vi "AlliGator FLI Dataset Series Actions.vi"(0 "AlliGator Q Elements":T4[](array[typedef]), 1 "VI in":refnum<vi>, 2 "Script in":bool, 5 "AlliGator IV DVR in":refnum<data-value>, 7 "AlliGator Q Event in":T5=enum."GUI:Idle", 9 "Data":variant, 11 "error in (no error)":errorcluster, 12 "AlliGator Ctrl Refnums":T6) -> (3 "Script out":bool, 4 "Alligator Queue Elements":T4[](array[typedef]), 6 "AlliGator IV DVR out":refnum<data-value>, 10 "[Notebook Message]":T1[](array[typedef]) {"Message Style"."Text Alignment" items=["Left", "Right", "Center"]}, 15 "error out":errorcluster)   [LabVIEW 2021, in "AlliGator Action Engine.lvlib"]
doc: "Processes AlliGator FLI Dataset Series-related actions."
uses:
  AlliGator Action Engine.lvlib
  AlliGator Internal Variables v2.ctl
  <vilib>/vision/Image Controls.llb/IMAQ Image.ctl
  AlliGator Gate Image Set.ctl
  AlliGator FLI Dataset Type.ctl
  AlliGator Data Series Type.ctl
  AlliGator Dataset Channel.ctl
  AlliGator Gate Arithmetic.ctl
  AlliGator Displayed Image.ctl
  Image/Named ROI Description.ctl
  AlliGator Decay Metadata v3.ctl
  AlliGator Decay Background Subtraction Info.ctl
  AlliGator Baseline Subtraction Method.ctl
  Graphs/XY Graph/XY Graph Plot Shift Parameters.ctl
  Graphs/XY Graph/XY Graph Plot Shift Method.ctl
  AlliGator Decay Extrapolation Parameters.ctl
  Phasor/Calibration Phasor (m, phi).ctl
  Phasor/Phasor Reference Series.ctl
  Phasor/Phasor Calibration Map v2.ctl
  Phasor/Phasor (g, s).ctl
  AlliGator Raw Phasor Plot Data v4.ctl
  Phasor/Phasor Standard Deviation Options.ctl
  AlliGator Phasor Multi-Harmonic Data.ctl
  Phasor/Phasor Harmonic Data.ctl
  AlliGator Decay Fit Options & Parameters v2.ctl
  Fits/IRF(X)PSED/Decay Fit Options v2.ctl
  Fits/Decay Convolution/Decay Model.ctl
  Fits/Residual Type.ctl
  Fits/IRF(X)PSED/Fit Weights Type.ctl
  Fits/Non-linear Fitting Method v2.ctl
  Fits/Fit Calculation Method.ctl
  Fits/Non-linear Fitting Algorithm.ctl
  AlliGator Decay Fit Parameter Constraints 2.ctl
  Fits/IRF(X)PSED/Decay Fit Parameters In List.ctl
  Fits/IRF(X)PSED/MLE Baseline Offset Type.ctl
  AlliGator Decay Preprocessing Parameters.ctl
  Fits/IRF(X)PSED/Decay Fit Parameters & Derived Quantities List.ctl
  AlliGator Q Event.ctl
  AlliGator Ctrl Refnums.ctl
  AlliGator Other Ctrl Refnums.ctl
  AlliGator State Indicator.ctl
  AlliGator Phasor Plot Ctrl Refnums.ctl
  AlliGator Phasor Graph Ctrl Refnums.ctl
  Phasor/Phasor Calibration Type.ctl
  AlliGator Dataset Ctrl Refnums.ctl
  AlliGator Registered Events Ctrl Refnums.ctl
  AlliGator Image Histogram Control Refnums.ctl
  Histograms/Linear Histogram Options.ctl
  Histograms/Histogram Bin Option.ctl
  Histograms/Histogram Bin Position.ctl
  AlliGator Decay Fit Map Control Refnums.ctl
  AlliGator Q Element.ctl
  Notebook/Notebook Message Object.ctl
  Rich Text Box/Text Formatting.ctl
  Rich Text Box/Text Colors.ctl
  Alligator Elements Order in Action Stack.ctl
  AlliGator Variables List.ctl
  AlliGator Series Analysis Type.ctl
  AlliGator Globals.vi
  Variant/Variant to Data/Variant to DBL.vi
  Variant/Variant to Data/Variant to Boolean.vi
  AlliGator Add Action Array to Stack.vi
  GUI/GUI.lvlib
  AlliGator Accumulated Dataset.lvlib
  AlliGator Scripts.lvlib
  Sound/Sound.lvlib
  AlliGator Decay Fit.lvlib
  AlliGator Internal Variables.lvlib
  Image/Image.lvlib
  Variant/Variant to Data/Variant to Data.lvlib
  AlliGator Source Image.lvlib
  AlliGator Globals, Variables & Constants.lvlib
  Rich Text Box/Rich Text Box.lvlib
  Phasor/Phasor.lvlib
  AlliGator Decay Preprocessing.lvlib
  Graphs/XY Graph/XY Graph Add-Ons.lvlib
  AlliGator Phasor Graph.lvlib
  AlliGator Files.lvlib
  AlliGator Phasor Plot.lvlib
  Fits/Fits.lvlib
  AlliGator Decay Fit Parameter Map.lvlib
  AlliGator Settings.lvlib
  AlliGator GUI.lvlib
  AlliGator Dual-Channel Datasets.lvlib
  Histograms/Histogram Window.lvlib
  Notebook/Notebook.lvlib
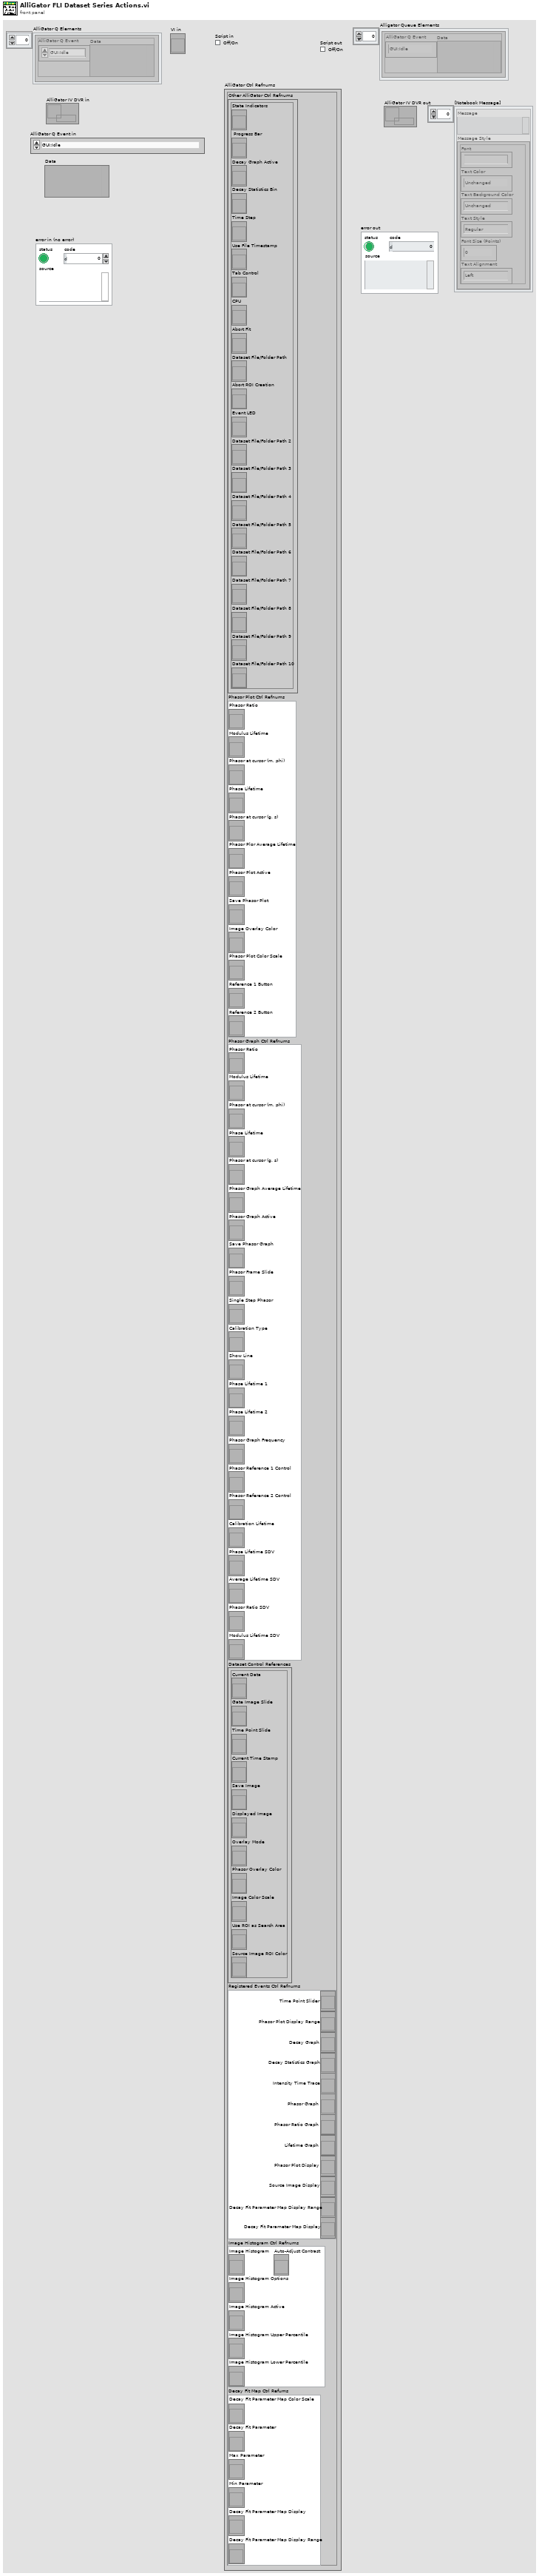
[diagram p1: front panel]
types:
  T1 = typedef "Notebook.lvlib/Notebook Message Object.ctl" = cluster{"Message":string, "Message Style":T2}
  T2 = typedef "Rich Text Box.lvlib/Text Formatting.ctl" = cluster{"Font":string, "Text Color":T3, "Text Background Color":T3, "Text Style":enum16{"Regular", "Bold", "Italic", "Underline", "Strikeout"}, "Font Size (Points)":dbl, "Text Alignment":i32}
  T3 = typedef "Rich Text Box.lvlib/Text Colors.ctl" = enum16{"Unchanged", "Black", "Blue", "Brown", "Gray", "Green", "Orange", "Pink", "Red", "White"}
  T4 = typedef "AlliGator Action Engine.lvlib/AlliGator Q Element.ctl" = cluster{"AlliGator Q Event":T5, "Data":variant}
  T5 = typedef "AlliGator Action Engine.lvlib/AlliGator Q Event.ctl" = enum16{"---- Files ----", "Files:Set Batch Export Files To Save", "Files:Set Dataset Loading & Pre-processing Options", "Files:Check #Frames in Dataset", "Files:Increment Frame Index", "Files:Open Mask Image", "Files:Open White Light Image", "Files:Open Single Dataset", "Files:New Folder of Folders Selected", "Files:Load File (all Types)_Scriptable", "Files:Move Flattened Series to Folders Series", "Files:Select Folder", "Files:Load FLI Dataset", "Files:Load Swiss SPAD 1 Dataset", "Files:Load Swiss SPAD 2 Dataset", "Files:Load .sdt FLI Dataset", "Files:Load .ptu FLI Dataset", "Files:Load .bin FLI Dataset", "Files:Load Single Gate Image Folder", "Files:Load I/m/phi Dataset (deprecated)", "Files:Load Single Image", "Files:Subtract Background File", "Files:Export FLI Dataset", "Files:Load HDF5 FLI Dataset", "Files:Set Destination File Path", "Files:Save Mask Image", "Files:Batch Conversion", "Files:New Folder Selected", "Files:Close FLI Dataset", "Files:Close FLI Dataset Series", "Files:Close White Light Image", "Files:Close Mask Image", "---- FLI Dataset ----", "FLI Dataset:Channel Arithmetic", "FLI Dataset:Export Average Lifetime Map as ASCII", "FLI Dataset:Export User-Defined Quantity Map as ASCII", "FLI Dataset:Python Function FLI Dataset Event", "FLI Dataset:ROI Analysis", "FLI Dataset:Tilted Logistic Square Gated IRF Characteristics Map", "FLI Dataset:Logistic Square Gated IRF Characteristics Map", "FLI Dataset:Square Gated IRF Characteristics Map", "FLI Dataset:Multi-ROI Single-Pixel Phasor Analysis", "FLI Dataset:Multi-ROI Single-Pixel NLSF Analysis", "FLI Dataset:All ROIs IRF Extraction", "FLI Dataset:All ROIs Decay Fit Non-Interactive (Fast + Individual IRF)", "FLI Dataset:All ROIs Phasor Analysis", "FLI Dataset:All ROIs Decay Fit", "FLI Dataset:Fluorescence Decay Statistics", "FLI Dataset:Update Decay Statistics Graph", "FLI Dataset:Get Decay from ROI", "FLI Dataset:All ROIs Average Lifetimes", "---- FLI Dataset Series ----", "FLI Dataset Series:Sum All Datasets in Series", "FLI Dataset Series:Add Dataset to Accumulated Dataset", "FLI Dataset Series:Display Accumulated Dataset", "FLI Dataset Series:Clear Dataset Series Sum", "FLI Dataset Series:Time-Series Analysis (NLSF)", "FLI Dataset Series:Time-Series Analysis (Phasor)", "---- Image ----", "Image:Update Image Profile Plots", "Image:Image Histogram Cursor Move", "Image:Image Histogram", "Image:Image Contrast", "Image:Set Image Histogram Cursor Move Flag", "Image:Clear Image Overlay", "Image:Use ROI as Search Area", "Image:Set ROI Diameter", "Image:Save Image Data as TIFF", "Image:Save Displayed Image with Overlay", "Image:Save Image Overlay Only", "Image:Save Image as Hot Pixel Mask", "Image:Change Source Image Color Palette", "Image:Copy Image to Clipboard", "Image:Source Image ROI Selection", "Image:Delete All ROIs", "Image:Delete All Unselected ROIs", "Image:Delete ROI", "Image:Merge All ROIs", "Image:Store ROI", "Image:Source Image ROI Storage", "Image:Export ROI Description to Notebook", "Image:Save ROI", "Image:Load ROI", "Image:Paste ROI Definition", "Image:Clear ROI", "Image:Identify ROIs in Mask Image", "Image:Create Complementary ROI", "Image:Create Contour ROI", "Image:Create ROI(s) from Pixels with Peak above Min_Scriptable", "Image:Create ROI(s) from Pixels with Intensity above Min_Scriptable", "Image:Compute ROI Statistics", "Image:Delete ROI(s) based on ROI Characteristics", "Image:Create ROI Grid", "Image:ROI to Individual Pixel ROIs", "Image:Python Function Source Image Event", "Image:Show Phasor Calibration Map ROI Centers", "Image:Convert ROI to Mask Image", "Image:Mouse Move", "Image:Mouse Up", "Image:Set Source Image Mouse Move Flag", "Image:Add Scale Bar Overlay", "Image:Delete Existing ROIs Option", "---- Decay ----", "Decay:Clear IRF/Reference Plot", "Decay:Clear Local IRFs", "Decay:Add Decay to Graph", "Decay:Smoothen Plot", "Decay:Smoothen Plot Tail", "Decay:Average Selected Plots", "Decay:Extract IRF", "Decay:Optimal IRF Extraction", "Decay:Threshold IRF", "Decay:Fit to Model IRF", "Decay:Fit IRF to Square Gate", "Decay:Fit IRF to Logistic Square Gate", "Decay:Fit IRF to Tilted Logistic Square Gate", "Decay:Create Bounding Cursors Set", "Decay:Export Bounding Cursors Definition to Notebook", "Decay:Denoise Plot", "Decay:Compute Cumulative Function", "Decay:Use as Reference Decay", "Decay:Show Reference Decay/IRF", "Decay:Extrapolate Decay", "Decay:Create Head & Tail Bounding Cursors", "Decay:Store Cursor-defined Head & Tail Fractions", "Decay:Rebin Plot", "Decay:1-Normalize Decay", "Decay:[0-1]-Normalize Plot", "Decay:Straighten Decay", "Decay:Shift Decay", "Decay:Fold Decay", "Decay:Fit Decay", "Decay:Global Fit of Selected Decays", "Decay:Post Global Fit Script", "Decay:Add Global Fit Parameters to Graph", "Decay:Add Decay Parameter(s) to Plot (Graph)", "Decay:Export Decay to Phasor Graph", "Decay:Plot Decay Shifts", "Decay:Compute Average Lifetime", "Decay:Plot Convolution", "Decay:Graph Tip Strip Update", "---- Decay Statistics ----", "Decay Statistics:Tip Strip Update", "---- Intensity Time Trace ----", "Intensity Time Trace:Use File Timestamp", "Intensity Time Trace:Load Intensity Corrections File", "Intensity Time Trace:Clear Intensity Corrections File", "Intensity Time Trace:Tip Strip Update", "---- Phasor Plot ----", "Phasor Plot:Build Phasor Plot", "Phasor Plot:Change Phasor Plot Color Palette", "Phasor Plot:Adjust Phasor Plot Display Range", "Phasor Plot:Highlight Image ROI in Phasor Plot", "Phasor Plot:Save Phasor Plot Image with Overlay", "Phasor Plot:Export Complex Phasor Map", "Phasor Plot:Export Phasor Ratio Map", "Phasor Plot:Export Average Lifetime Map", "Phasor Plot:Compute Phase Lifetime Histogram", "Phasor Plot:Compute Phasor Ratio Histogram", "Phasor Plot:Compute Phase Lifetime vs Intensity Scatter Plot", "Phasor Plot:Weber 2-Component Decomposition", "Phasor Plot:Update Phasor Color Map Vertices", "Phasor Plot:Clear Phasor Overlay", "Phasor Plot:Use Segment Extremities as References", "Phasor Plot:Use UC/Segment Intersections as References", "Phasor Plot:Use UC/Principal Axis Intersections as References", "Phasor Plot:Use UC/Linear Fit Intersections as References", "Phasor Plot:Update Phasor Plot Reference", "Phasor Plot:Show Local Phasor Info in Phasor Plot", "Phasor Plot:Update Phasor Plot State", "Phasor Plot:Phasor Plot ROI Storage", "Phasor Plot:Phasor Plot ROI Selection", "Phasor Plot:Python Function Phasor Plot Event", "Phasor Plot:Overlay Phasor ROI, Ratio or Map in Source Image", "Phasor Plot:Compute Decay of Selected Phasors", "Phasor Plot:Phasor at Image Pixel", "Phasor Plot:Mouse Move", "Phasor Plot:Mouse Up", "Phasor Plot:Display Range Mouse Move", "Phasor Plot:Set Mouse Move Flag", "---- Phasor Graph ----", "Phasor Graph:Calibrated Phasor Map Series", "Phasor Graph:Whole Image Phasor Scatter Plot (Todo)", "Phasor Graph:Get Phasor Value", "Phasor Graph:Create New Phasor Plot Dialog", "Phasor Graph:Update Last Phasor Value", "Phasor Graph:Update Phasor (m, phi)", "Phasor Graph:Remove Single Phasor from Plot", "Phasor Graph:Add Single Phasor to Plot", "Phasor Graph:Remove Phasor Plot", "Phasor Graph:Remove Selected Phasor Plots", "Phasor Graph:Clear Phasor Data", "Phasor Graph:Clear Phasor Graph", "Phasor Graph:Cursor Move", "Phasor Graph:Draw Cursor Connecting Line", "Phasor Graph:Clear Cursor Connecting Line", "Phasor Graph:Find UC Intersection", "Phasor Graph:Use UC/Cursor-Defined Line Intersections", "Phasor Graph:Use Selected Plots Fitted Line/UC Intersections", "Phasor Graph:Use Selected Plots Principal Axis/UC Intersections", "Phasor Graph:Show Single Phasor", "Phasor Graph:Save Single Phasor Plot", "Phasor Graph:Save All Phasor Plots", "Phasor Graph:Load Phasor Plot(s)", "Phasor Graph:Phasor Multiplication", "Phasor Graph:Compute Average Phasor", "Phasor Graph:Compute Multiple Average Phasors (Selected Plots)", "Phasor Graph:Export Single Phasor Plot Phase Lifetimes", "Phasor Graph:Phase Lifetime Trajectory", "Phasor Graph:Phase Lifetime vs Intensity Scatter Plot (deprecated)", "Phasor Graph:Parameter 2 vs Parameter 1 Scatter Plot", "Phasor Graph:Use Cursor n Location", "Phasor Graph:Set Reference n to Current Phase Lifetime Value", "Phasor Graph:Set Reference n to Lifetime Value", "Phasor Graph:Set Cursor n Location", "Phasor Graph:Save Phasor Graph Image", "Phasor Graph:Update SEPL Plot", "Phasor Graph:Export Single Phasor Plot Data", "Phasor Graph:Export Selected Phasor Plots Data", "Phasor Graph:Python Function Phasor Graph Event", "Phasor Graph:Tip Strip Update", "---- Calibration ----", "Calibration:Set Calibration Type", "Calibration:Load/Save Phasor Calibration", "Calibration:Load/Save Phasor Calibration Series", "Calibration:Load/Save Phasor Calibration Map", "Calibration:Use as Calibration", "Calibration:Compute Optimal Calibration from Phasor References", "Calibration:Clear Phasor Calibration", "Calibration:Single Phasor Calibration Information", "Calibration:Use as Calibration Series", "Calibration:Use as Calibration Map", "Calibration:Clear Calibration Series", "Calibration:Phasor Calibration Series Information", "Calibration:Clear Calibration Map", "Calibration:Phasor Calibration Map Information", "Calibration:Apply Phasor Calibration", "Calibration:Update Single Plot Calibration", "Calibration:Update Multiple Plots Calibration", "Calibration:Clear Single Plot Calibration", "Calibration:Clear All Plots Calibrations", "Calibration:Clear Plot(s) Calibration(s)?", "Calibration:Phasor Calibration Maps (# Gates Series)", "---- Phasor Ratio ----", "Phasor Ratio:Clear Reference n", "Phasor Ratio:Toggle Selected Plot(s)  Lock to Reference 1", "Phasor Ratio:Use as Reference n", "Phasor Ratio:Send Reference n to Notebook", "Phasor Ratio:Toggle Selected Plot(s)  Lock to Reference 2", "Phasor Ratio:Compute Phasor Ratio at Mouse Location", "Phasor Ratio:Compute Phasor Plot's Average Phasor Ratio", "Phasor Ratio:Compute Time-Series Phasor Ratios", "Phasor Ratio:Fit Line to Phasor Ratio Plot", "Phasor Ratio:Save References", "Phasor Ratio:Load References", "Phasor Ratio:Update Phasor Reference 1", "Phasor Ratio:Update Phasor Reference 2", "Phasor Ratio:Move Cursor n to Reference n", "Phasor Ratio:Use as Phasor Reference 1 Lifetime", "Phasor Ratio:Use as Phasor Reference 2 Lifetime", "Phasor Ratio:Export Phasor Ratio Map as ASCII", "Phasor Ratio:Tip Strip Update", "---- Lifetime & Other Parameters Graph ----", "Lifetime:Tip Strip Update", "---- Decay Fit Parameter Map ----", "Decay Fit Parameter Map:Export ROI NLSF Data as ASCII", "Decay Fit Parameter Map:Set Decay Fit  Parameter Map Selection", "Decay Fit Parameter Map:Build Decay Fit Parameter Map", "Decay Fit Parameter Map:Change Decay Fit Parameter Map Color Palette", "Decay Fit Parameter Map:Export Decay Fit Parameter Map Data as ASCII", "Decay Fit Parameter Map:Export All Decay Fit Parameter Maps Data as ASCII", "Decay Fit Parameter Map:Send Map Data to Lifetime Graph", "Decay Fit Parameter Map:Save Decay Fit Parameter Map Image", "Decay Fit Parameter Map:Save-Load IRFs & Fit Data", "Decay Fit Parameter Map:Update Local Decay Plots", "Decay Fit Parameter Map:Python Function Decay Fit Parameters Map Event", "Decay Fit Parameter Map:Overlay Decay Fit Parameter Map in Source Image", "Decay Fit Parameter Map:Plot Map Data vs Intensity", "Decay Fit Parameter Map:Mouse Up", "Decay Fit Parameter Map:Display Range Mouse Move", "---- Generic Graph ----", "Generic Graph:Generic XY Graph Event", "Generic Graph:Python Function XY Graph Event", "Generic Graph:New Plot", "Generic Graph:Save Plot", "Generic Graph:XY Plot Histogram", "Generic Graph:Set XY Graph Plot Name", "Generic Graph:Set Last Cursor Style", "Generic Graph:Tip Strip Update", "---- GUI ----", "GUI:Start Script", "GUI:Type of Displayed Image Changed", "GUI:Gate Image Slide Changed", "GUI:Show Busy Icon", "GUI:Show Busy Icon & Abort Button", "GUI:Hide Busy Icon", "GUI:Hide Busy Icon & Abort Button", "GUI:Abort", "GUI:End Script", "GUI:Start Timing", "GUI:End Timing", "GUI:Set State Indicator", "GUI:Send Parameters JSON Strings to Clipboard", "GUI:Set Gate Step", "GUI:Idle", "GUI:Initialization", "GUI:Quit", "GUI:Increment Dataset Index", "GUI:Set Dataset Index to -1", "GUI:Time Series Slider Moved", "GUI:Time Series Slider Changed", "GUI:Toggle Playback or Loop", "GUI:Playback Script", "GUI:Set Phasor Frequency", "GUI:Open Window", "GUI:Start Test Script", "GUI:End Test Script", "DEBUG"}
  T6 = typedef "AlliGator GUI.lvlib/AlliGator Ctrl Refnums.ctl" = cluster{"Other AlliGator Ctrl Refnums":T7, "Phasor Plot Ctrl Refnums":T8, "Phasor Graph Ctrl Refnums":T9, "Dataset Control References":T10, "Registered Events Ctrl Refnums":T11, "Image Histogram Ctrl Refnums":T12, "Decay Fit Map Ctrl Refums":T13}
  T7 = typedef "AlliGator GUI.lvlib/AlliGator Other Ctrl Refnums.ctl" = cluster{"State Indicators":refnum<vi>, " Progress Bar":refnum<vi>, "Decay Graph Active":refnum<vi>, "Decay Statistics Bin":refnum<vi>, "Time Step":refnum<vi>, "Use File Timestamp":refnum<vi>, "Tab Control":refnum<vi>, "CPU":refnum<vi>, "Abort Fit":refnum<vi>, "Dataset File/Folder Path":refnum<vi>, "Abort ROI Creation":refnum<vi>, "Event LED":refnum<vi>, "Dataset File/Folder Path 2":refnum<vi>, "Dataset File/Folder Path 3":refnum<vi>, "Dataset File/Folder Path 4":refnum<vi>, "Dataset File/Folder Path 5":refnum<vi>, "Dataset File/Folder Path 6":refnum<vi>, "Dataset File/Folder Path 7":refnum<vi>, "Dataset File/Folder Path 8":refnum<vi>, "Dataset File/Folder Path 9":refnum<vi>, "Dataset File/Folder Path 10":refnum<vi>}
  T8 = typedef "AlliGator GUI.lvlib/AlliGator Phasor Plot Ctrl Refnums.ctl" = cluster{"Phasor Ratio":refnum<vi>, "Modulus Lifetime":refnum<vi>, "Phasor at cursor (m, phi)":refnum<vi>, "Phase Lifetime":refnum<vi>, "Phasor at cursor (g, s)":refnum<vi>, "Phasor Plor Average Lifetime":refnum<vi>, "Phasor Plot Active":refnum<vi>, "Save Phasor Plot":refnum<vi>, "Image Overlay Color":refnum<vi>, "Phasor Plot Color Scale":refnum<vi>, "Reference 1 Button":refnum<vi>, "Reference 2 Button":refnum<vi>}
  T9 = typedef "AlliGator GUI.lvlib/AlliGator Phasor Graph Ctrl Refnums.ctl" = cluster{"Phasor Ratio":refnum<vi>, "Modulus Lifetime":refnum<vi>, "Phasor at cursor (m, phi)":refnum<vi>, "Phase Lifetime":refnum<vi>, "Phasor at cursor (g, s)":refnum<vi>, "Phasor Graph Average Lifetime":refnum<vi>, "Phasor Graph Active":refnum<vi>, "Save Phasor Graph":refnum<vi>, "Phasor Frame Slide":refnum<vi>, "Single Step Phasor":refnum<vi>, "Calibration Type":refnum<vi>, "Show Line":refnum<vi>, "Phase Lifetime 1":refnum<vi>, "Phase Lifetime 2":refnum<vi>, "Phasor Graph Frequency":refnum<vi>, "Phasor Reference 1 Control":refnum<vi>, "Phasor Reference 2 Control":refnum<vi>, "Calibration Lifetime":refnum<vi>, "Phase Lifetime SDV":refnum<vi>, "Average Lifetime SDV":refnum<vi>, "Phasor Ratio SDV":refnum<vi>, "Modulus Lifetime SDV":refnum<vi>}
  T10 = typedef "AlliGator GUI.lvlib/AlliGator Dataset Ctrl Refnums.ctl" = cluster{"Current Data":refnum<vi>, "Gate Image Slide":refnum<vi>, "Time Point Slide":refnum<vi>, "Current Time Stamp":refnum<vi>, "Save Image":refnum<vi>, "Displayed Image":refnum<vi>, "Overlay Mode":refnum<vi>, "Phasor Overlay Color":refnum<vi>, "Image Color Scale":refnum<vi>, "Use ROI as Search Area":refnum<vi>, "Source Image ROI Color":refnum<vi>}
  T11 = typedef "AlliGator GUI.lvlib/AlliGator Registered Events Ctrl Refnums.ctl" = cluster{"Time Point Slider":refnum<vi>, "Phasor Plot Display Range":refnum<vi>, "Decay Graph":refnum<vi>, "Decay Statistics Graph":refnum<vi>, "Intensity Time Trace":refnum<vi>, "Phasor Graph":refnum<vi>, "Phasor Ratio Graph":refnum<vi>, "Lifetime Graph":refnum<vi>, "Phasor Plot Display":refnum<vi>, "Source Image Display":refnum<vi>, "Decay Fit Parameter Map Display Range":refnum<vi>, "Decay Fit Parameter Map Display":refnum<vi>}
  T12 = typedef "AlliGator GUI.lvlib/AlliGator Image Histogram Control Refnums.ctl" = cluster{"Image Histogram":refnum<vi>, "Image Histogram Options":refnum<vi>, "Image Histogram Active":refnum<vi>, "Image Histogram Upper Percentile":refnum<vi>, "Image Histogram Lower Percentile":refnum<vi>, "Auto-Adjust Contrast":refnum<vi>}
  T13 = typedef "AlliGator Decay Fit Parameter Map.lvlib/AlliGator Decay Fit Map Control Refnums.ctl" = cluster{"Decay Fit Parameter Map Color Scale":refnum<vi>, "Decay Fit Parameter":refnum<vi>, "Max Parameter":refnum<vi>, "Min Parameter":refnum<vi>, "Decay Fit Parameter Map Display":refnum<vi>, "Decay Fit Parameter Map Display Range":refnum<vi>}
  T14 = typedef "AlliGator Globals, Variables & Constants.lvlib/AlliGator Variables List.ctl" = enum16{"---- GUI ----", "Initialization Status", "State Indicators Refnum", "Original AlliGator Menu Items", "Current Action Loop State", "Script in progress", "Playback", "Loop Playback", "Search ROI Used", "Search ROI", "Decay Graph Max Legend Size", "Intensity Graph Max Legend Size", "Decay Statistics Graph Max Legend Size", "Phasor Graph Max Legend Size", "Phasor Ratio Graph Max Legend Size", "Lifetime Graph Max Legend Size", "---- Files ----", "Export Dataset Frames as Individual Files", "Show Batch Export Help Balloons", "Frames in Dataset", "ptu File Frame Start Indices", "Current Frame in Dataset", "Current Frame Timestamp", "------ Python Plugins ------", "Python Plugins Information", "Python Session", "Valid Python Session?", "---- Source Image ----", "Dataset Loaded", "Dataset Metadata", "Dataset Channel", "Dataset Data Description", "Background Dataset Metadata", "Background Dataset Channel", "Background Dataset Data Description", "Background File Subtraction", "Background File Path", "Background File Pile-up Correction", "Background File Pixel Well Capacity", "Background File Scaling Factor", "Source Image ROIs", "Current Source Image ROI", "Source Image ROI Event Refnum", "X_Source Image Display Range", "X_Source Image Palette Information", "Source Image Palette List", "Source Image Scale", "Current Dataset Load Settings", "Source Image:ROI Overlay Color", "---- Image Profile Window ----", "Image Profile:Overlay ROI in Source Image", "Image Profile Window Event Refnum", "Image Profile:IntensityType", "Image Profile:Intensity Average Type", "Image Profile:Intensity-weighted SDV", "Image Profile:Box Profile Type", "Image Profile Window Open", "Image Profile:Plotted Fit Parameter", "X_Type of Displayed Image", "X_Time Gate Slider", "Dataset Path", "Source Image Overlay to Erase", "Is Displayed Image Accumulated", "White Light Image Modified", "Mask Image Modified", "Macrotime Gate Separation", "------ Phasor Graph -------", "Phasor Graph:Show Line", "---- Phasor Plot ---", "Phasor Plot Parameters Changed", "FLI Dataset Modified since last Phasor Plot Calculation", "Phasor Harmonics Data", "Selected Phasor Harmonics", "Phasor Harmonic Manager Event Refnum", "Phasor Plot ROIs", "Current Phasor Plot ROI", "Phasor Plot ROI Event Refnum", "Phasor Plot Image Reference Points", "Phasor Plot Computed", "Phasor Plot Palette Information", "Phasor Plot Palette List", "Phasor Ratio Palette Information", "Phasor Ratio Palette List", "Phasor Image Scale", "Phasor Plot Image Overlay to Erase", "Phasor Plot Image Elements to Update", "Current Phasor Plot Calculation Parameters", "Current Phasor Calibration Options", "Reset Cumulated Phasor Plot", "Phasor Ratio Reference 1", "Phasor Ratio Lifetime Reference 1", "Phasor Ratio Reference 1 Frequency", "Phasor Ratio Reference 2", "Phasor Ratio Lifetime Reference 2", "Phasor Ratio Reference 2 Frequency", "---- Decay Analysis ----", "Number of Selected Decays to Fit", "LS Fit Results", "LAR Fit Results", "BS Fit Results", "Last Decay Max - Min", "Best Fit Parameters", "Best Fit Parameter Names", "Actual Size X", "Actual Size Y", "Binning X", "Binning Y", "Actual # Gates", "Dataset Number", "Gates to...", "Gates Skipped", "Gates to keep", "Gate Step", "Gate Separation", "Reversed Gates", "Pile-up Correction", "Pixel Well Capacity", "Background Subtracted", "Background Subtraction Method", "Background Definition Range", "Background File (deprecated)", "Number of Dataset Accumulated", "Array of Accumulated Dataset Paths", "Do Averaged Datasets", "Destination File Path", "Process Plot Target", "Use 1/D as Phasor Frequency", "---- Decay Fit Parameter Map -----", "Decay Fit Parameter Map Palette Information", "Decay Fit Parameter Map Palette List", "Local Decay Graph Window Event Refnum", "------- Local Decay Window ---------", "Use normalized IRF for convolution", "----- Miscellaneous ----", "Skippable Dialog Windows Status"}
  T15 = typedef "AlliGator Action Engine.lvlib/Alligator Elements Order in Action Stack.ctl" = enum16{"Enqueue 2 AFTER 1", "Enqueue 2 BEFORE 1"}
  T16 = typedef "AlliGator Scripts.lvlib/AlliGator Series Analysis Type.ctl" = enum16{"Current ROI (Fixed)", "All ROIs (Fixed)", "Sequential ROIs"}
  T17 = typedef "AlliGator Internal Variables.lvlib/AlliGator Internal Variables v2.ctl" = cluster{"Displayed Image":T18, "White Light Image":T18, "Mask Image":T18, "ROI Mask Image":T18, "Current Dataset Images 1":T19, "Background Dataset Images 1":T19, "Current Dataset Images 2":T19, "Background Dataset Images 2":T19, "Current Dataset Arithmetic Images":T19, "Accumulated Dataset Images 1":T19, "Accumulated Dataset Images 2":T19, "Accumulated Dataset Arithmetic Images":T19, "Phasor Plot Image":T18, "Decay Fit Parameter Map Image":T18, "Single Data Point Path":path, "White Light Image Path":path, "Mask Image Path":path, "Time-Series Folder":path, "[Time-Series Paths]":path[], "Current Dataset":i32, "Single Dataset Type":T20, "Current Folder":string, "AlliGator Data Series Type":T21, "# Datasets":i32, "Dual-Channel Dataset":bool, "Selected Channel Name":string, "Dataset Channel":T22, "Channel Arithmetic":T23, "Dual-Channel Background Dataset":bool, "Background Channel":T22, "Dual-Channel Accumulated Dataset":bool, "Start Time":dbl, "[Time-Series Timestamps]":dbl[], "[Intensity Corrections]":dbl[], "Time Series Script":bool, "Type of Displayed Image":T24, "Gate Image Slide":u16, "# Gates":i32, "ROIs":T25[], "ROI Decay":cluster{"t Array":dbl[], "I Array":dbl[]}, "Valid Decay":bool, "Decay  Metadata":T27, "Reference Decay Plot Name":string, "Reference Decay":cluster{"t Array":dbl[], "I Array":dbl[]}, "Decay Shift Plot":cluster{"Time Stamps":dbl[], "Decay Shifts":dbl[]}, "[Decays Max Values]":sgl[], "[Decays Min Values]":sgl[], "Calibration Phasor":T33, "Calibration Phasor Series":T34, "Phasor Calibration Map":T35, "Calibration Map MD5 Digest":string, "Last Raw Phasor":T36, "Last Calibrated Phasor":T36, "Last Calibrated Phasor SDV":T36, "Phasor Graph:Phasor Plot":cluster{"g Array":dbl[], "s Array":dbl[]}, "Phasor Graph:Phasor SDV Plot":cluster{"g Array":dbl[], "s Array":dbl[]}, "[Phasor Graph:Raw Phasor Plots]":T37[], "Phasor Plot locked to Ref 1":i32, "[Phasor Plot(s) locked to Ref 1]":i32[], "[Phasor Plot(s) locked to Ref 2]":i32[], "[Pixel Phasors]":T36[], "[[Sum Image]]":dbl[][], "[[CSG Phasors]]":csg[][], "[[Valid Pixel?]]":bool[][], "I/m/phi Dataset":cluster{"I/m/phi Dataset?":bool, "Base Frequency":dbl[unit], "Harmonic Orders":u8[]}, "Multi Phasor Plot Data":T39, "Decay Fit Options & Parameters":T41, "Fit Options: Decay Preprocessing Parameters":T52, "Fit Options: Reference Decay":cluster{"t Array":dbl[], "I Array":dbl[]}, "Is Full Image Parameters Map":bool, "Is Single-Pixels Parameters Map":bool, "NLSF Parameters Map X Resolution":i32, "NLSF Parameters Map Y Resolution":i32, "[Single Decay Fit Parameters]":dbl[], "Fit Model":T43, "[[Multiple Decays Fit Parameters]]":dbl[][], "[[Multiple Decays Fit Parameter SDVs]]":dbl[][], "[[IRFs]]":dbl[][], "IRF Array Time Axis":dbl[], "Decay Array Time Axis":dbl[], "[Decay Fit Parameter Names]":T53[], "[[Phasor Ratios]]":dbl[][], "[[Average Lifetimes]]":dbl[][], "Amplitude Weighted Average Lifetime":bool, "[Decay Sum]":dbl[], "[[User-defined Quantities]]":dbl[][], "User-defined Quantity":string}
  T18 = typedef "IMAQ Image.ctl" = refnum<image>
  T19 = typedef "AlliGator Internal Variables.lvlib/AlliGator Gate Image Set.ctl" = cluster{"SGL Image Max":T18, "SGL Image Sum":T18, "SGL Gate Images":T18[], "SGL Image Min":T18}
  T20 = typedef "AlliGator Files.lvlib/AlliGator FLI Dataset Type.ctl" = enum16{"HDF5 FLI Dataset", "Gate Image Folder", ".sdt FLI Dataset (Becker & Hickl)", ".ptu FLI Dataset (PicoQuant)", "SS1 FLI Dataset", "SS2 FLI Dataset", "I/m/phi Dataset", ".bin FLI Dataset (PicoQuant Binned)", ".bin FLI Dataset (Piccolo Binned)"}
  T21 = typedef "AlliGator Files.lvlib/AlliGator Data Series Type.ctl" = enum16{"Not a Supported Series", "Gate Images Folder Series", "SwissSPAD 2 Dataset Series", "B&H FLI Dataset Series", "PicoQuant PTU FLI Dataset Series", "PicoQuant BIN FLI Dataset Series", "Piccolo hist BIN FLI Dataset Series", "HDF5 FLI Dataset Series"}
  T22 = typedef "AlliGator Dual-Channel Datasets.lvlib/AlliGator Dataset Channel.ctl" = enum16{"G2", "INT"}
  T23 = typedef "AlliGator Settings.lvlib/AlliGator Gate Arithmetic.ctl" = enum16{"None", "INT-G2", "G2/INT*<INT>", "(1 - G2/INT)*<INT>"}
  T24 = typedef "AlliGator Source Image.lvlib/AlliGator Displayed Image.ctl" = enum16{"Single Gate", "Sum of All Gates", "Max of All Gates", "Min of All Gates", "-", "White Ligth Image", "Mask Image"}
  T25 = typedef "Image.lvlib/Named ROI Description.ctl" = cluster{"ROI Descriptor":T26, "ROI Name":string, "Overlay Color":u32}
  T26 = typedef "ROI Descriptor" = cluster{"Global Rectangle":i32[], "Contours":cluster{"ID":enum32{"External", "Internal"}, "Type":u32, "Coordinates":i32[]}[]}
  T27 = typedef "AlliGator Phasor Graph.lvlib/AlliGator Decay Metadata v3.ctl" = cluster{"ROI Descriptor":T26, "ROI Center":cluster{"X":i32, "Y":i32}, "Decay Background Subtraction Info":T28, "Decay Reverted":bool, "Decay Smoothened":bool, "Decay Straightened":bool, "Fitted Tau (Decay Straightening)":dbl, "Decay Shift Parameters":T30, "Decay Shifted":bool, "Decay Extrapolated":bool, "Decay Extrapolation Parameters":T32, "Decay Normalized":bool, "Fold Decay":bool, "# Folds":u32}
  T28 = typedef "AlliGator Decay Analysis.lvlib/AlliGator Decay Preprocessing.lvlib/AlliGator Decay Background Subtraction Info.ctl" = cluster{"Laser Period":dbl[unit], "Gate Duration":dbl[unit], "Baseline Subtraction Method":T29, "Background Definition Range":cluster{"Min Gate":dbl[unit], "Max Gate":dbl[unit]}, "Total Intensity w/o Bkgd Subtraction":dbl, "Bkgd-subtracted Intensity (exp)":dbl, "# Data Points":i32, "Background/Gate":dbl, "Fitted Lifetime":dbl[unit], "Bkgd-subtracted Intensity (theo)":dbl}
  T29 = typedef "AlliGator Decay Analysis.lvlib/AlliGator Decay Preprocessing.lvlib/AlliGator Baseline Subtraction Method.ctl" = enum16{"Mean", "Min", "Square Gated Single-Exponential", "File", "Constant"}
  T30 = typedef "XY Graph Add-Ons.lvlib/XY Graph Plot Shift Parameters.ctl" = cluster{"Type":T31, "Shift":dbl[unit], "Threshold":dbl, "Rotate":bool}
  T31 = typedef "XY Graph Add-Ons.lvlib/XY Graph Plot Shift Method.ctl" = enum16{"Default", "CFD", "Threshold", "Cross-Correlation"}
  T32 = typedef "AlliGator Decay Analysis.lvlib/AlliGator Decay Preprocessing.lvlib/AlliGator Decay Extrapolation Parameters.ctl" = cluster{"Additional Points":u32, "Head Fraction":dbl, "Fitted Tau":dbl, "Use Periodicity":bool, "Use Cursors":bool, "Tail Fraction":dbl}
  T33 = typedef "Phasor.lvlib/Calibration Phasor (m, phi).ctl" = cluster{"m":dbl, "phi":dbl, "Phasor Frequency":dbl[unit], "Reference Lifetime":dbl[unit]}
  T34 = typedef "Phasor.lvlib/Phasor Reference Series.ctl" = cluster{"m Array":dbl[], "phi Array":dbl[], "Phasor Frequency":dbl[unit], "Calibration Lifetime":dbl[unit]}
  T35 = typedef "Phasor.lvlib/Phasor Calibration Map v2.ctl" = cluster{"Phasor Frequency":dbl[unit], "Calibration Lifetime":dbl[unit], "ROI Centers":cluster{"X":i32, "Y":i32}[], "ROI Descriptors":T26[], "Map Resolution X":i32, "Map Resolution Y":i32, "z Array":cdb[]}
  T36 = typedef "Phasor.lvlib/Phasor (g, s).ctl" = cluster{"g":dbl, "s":dbl}
  T37 = typedef "AlliGator Phasor Graph.lvlib/AlliGator Raw Phasor Plot Data v4.ctl" = cluster{"Phasor Plot Name":string, "Raw Phasor Plot":T36[], "Phasor Frequency":dbl[unit], "[Decay Metadata]":T27[], "Raw Phasor Plot SDV":T36[], "Phasor SDV Options":T38, "[Calibration Phasor]":T33[]}
  T38 = typedef "Phasor.lvlib/Phasor Standard Deviation Options.ctl" = cluster{"Compute Estimated SDV":bool, "# Replicas":u32, "Use Estimated Average Phasor":bool}
  T39 = typedef "AlliGator Phasor Plot.lvlib/AlliGator Phasor Multi-Harmonic Data.ctl" = cluster{"Base Frequency":dbl[unit], "# Harmonics":u8, "Harmonic Orders":u8[], "Phasor Plot Settings Checksum":u64, "Phasor Harmonic Data Array":T40[]}
  T40 = typedef "Phasor.lvlib/Phasor Harmonic Data.ctl" = cluster{"Phasor Harmonic Name":string, "Phasor Plot Settings Checksum":u64, "Phasor Frequency":dbl[unit], "Base Frequency":dbl[unit], "Harmonic Order":u8, "Phasor Plot Parameters":string, "Phasor Array [[CSG]]":csg[][], "Dataset File Path":path}
  T41 = typedef "AlliGator Decay Fit Parameter Map.lvlib/AlliGator Decay Fit Options & Parameters v2.ctl" = cluster{"SYNC Period":dbl[unit], "Fit Options":T42, "Fit Parameter Constraints":T49[], "MLE Baseline Offset":dbl, "MLE Baseline Offset Type":T51}
  T42 = typedef "Fits.lvlib/Decay Fit Options v2.ctl" = cluster{"Show Fit Residuals":bool, "Fit Model":T43, "Residual Type":T44, "Max Decay Percentile":dbl, "Min Decay Percentile":dbl, "Show Full Decay":bool, "Weights":T45, "Fitting Method":T46, "Compute Parameter Uncertainties":bool, "Periodic Boundaries":bool, "Model Calculation":T47, "Period":dbl[unit], "Termination Criteria":cluster{"Max Iterations":i32, "Max Function Calls":i32, "Max Time":dbl[unit], "Function Tolerance":dbl, "Parameter Tolerance":dbl, "Gradient Tolerance":dbl, "Min Lambda":dbl, "Max Lambda":dbl, "Initial Tick Count":u32}, "Offset Resolution":dbl[unit], "Use Local IRF":bool, "Fitting Algorithm":T48}
  T43 = typedef "Fits.lvlib/Decay Model.ctl" = enum16{"1-Exponential", "2-Exponentials"}
  T44 = typedef "Fits.lvlib/Residual Type.ctl" = enum16{"Standard", "Normalized", "Reduced"}
  T45 = typedef "Fits.lvlib/Fit Weights Type.ctl" = enum16{"Unweighted", "1/Variance", "Best of All"}
  T46 = typedef "Fits.lvlib/Non-linear Fitting Method v2.ctl" = enum16{"Least Square", "Least Absolute Residual", "Bisquare", "MLE", "-", "Best of All"}
  T47 = typedef "Fits.lvlib/Fit Calculation Method.ctl" = enum16{"Simulation", "Convolution", "Integration"}
  T48 = typedef "Fits.lvlib/Non-linear Fitting Algorithm.ctl" = enum16{"Levenberg-Marquardt", "Trust-Region Dogleg"}
  T49 = typedef "AlliGator Decay Analysis.lvlib/AlliGator Decay Fit.lvlib/AlliGator Decay Fit Parameter Constraints 2.ctl" = cluster{"Fit Parameter":T50, "Min Value":dbl, "Max Value":dbl, "Global":bool, "Used":bool}
  T50 = typedef "Fits.lvlib/Decay Fit Parameters In List.ctl" = enum16{"Offset", "Baseline", "A_1", "tau_1", "A_2", "tau_2"}
  T51 = typedef "Fits.lvlib/MLE Baseline Offset Type.ctl" = enum32{"Absolute", "Percentage"}
  T52 = typedef "AlliGator Decay Analysis.lvlib/AlliGator Decay Preprocessing.lvlib/AlliGator Decay Preprocessing Parameters.ctl" = cluster{"Background Subtraction":bool, "Straighten Decay":bool, "Reverse Gates":bool, "1-Normalized Decay":bool, "Smoothen Decay":bool, "Smoothing Parameter":dbl, "Shift Decay":bool, "Decay Shift Parameters":T30, "Extrapolate Decay":bool, "Additional Points":u32, "Head Fraction":dbl, "Pixel-Normalize Decay":bool, "Use Periodicity":bool, "Use Cursors":bool, "Tail Fraction":dbl, "Use Decay Pre-Processing":bool, "Fold Decay":bool, "# Folds":u32, "[0-1]-Normalized Decay":bool}
  T53 = typedef "Fits.lvlib/Decay Fit Parameters & Derived Quantities List.ctl" = enum16{"Offset", "Baseline", "A_1", "tau_1", "A_2", "tau_2", "<tau>_a", "f1_a", "f2_a", "<tau>_i", "f1_i", "f2_i", "-", "R^2", "Chi^2"}
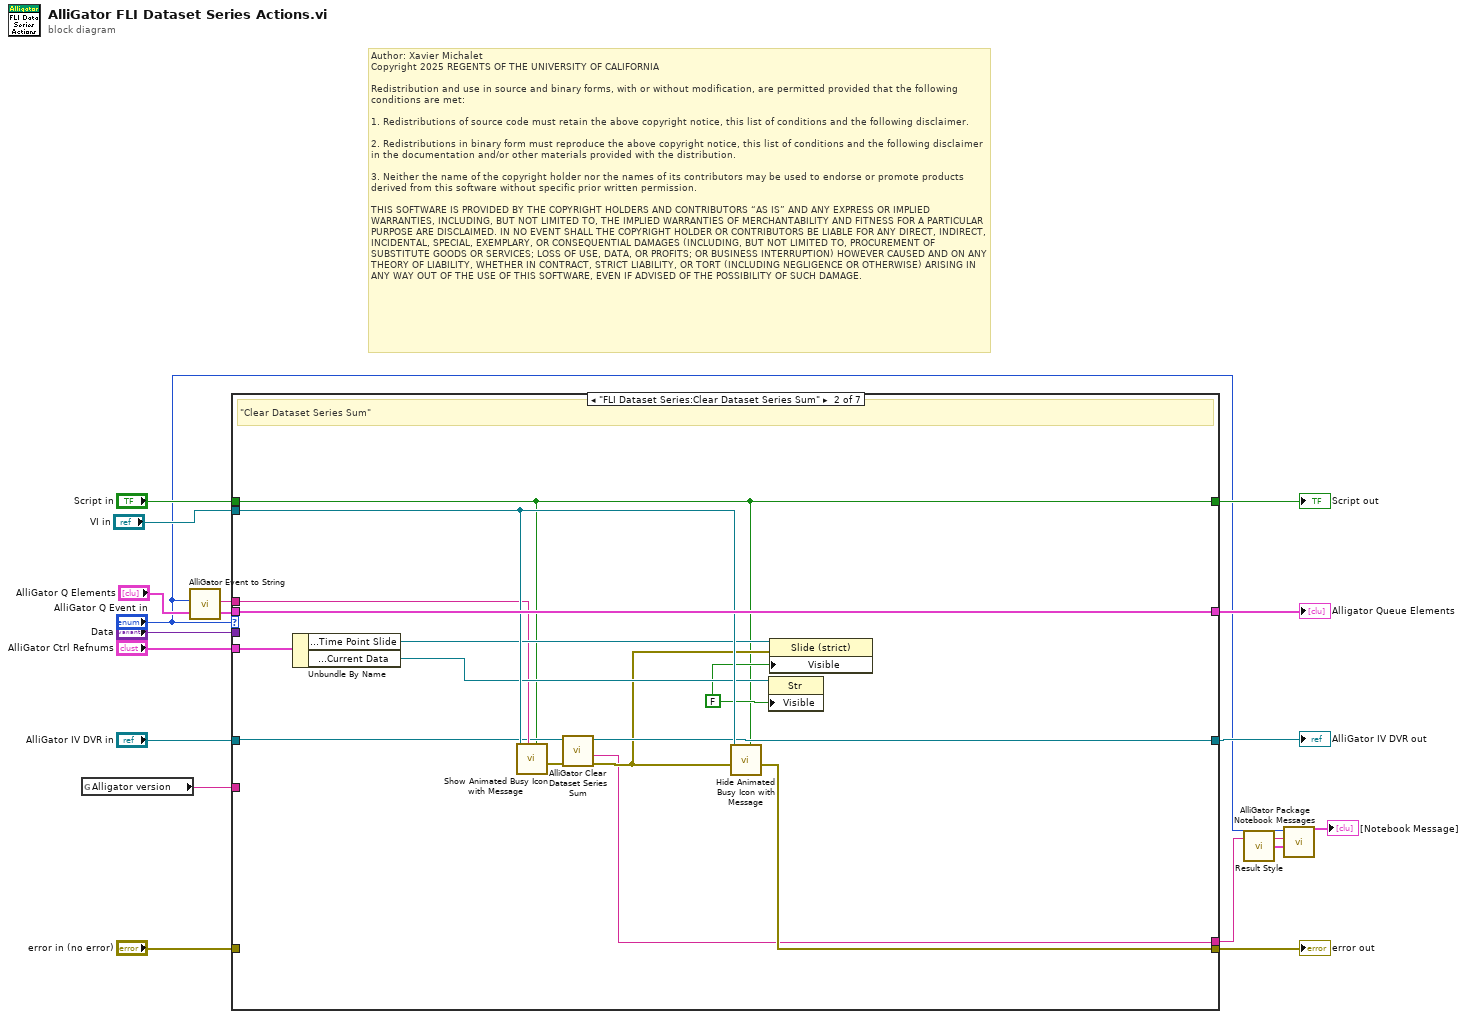
[diagram p0: block diagram]
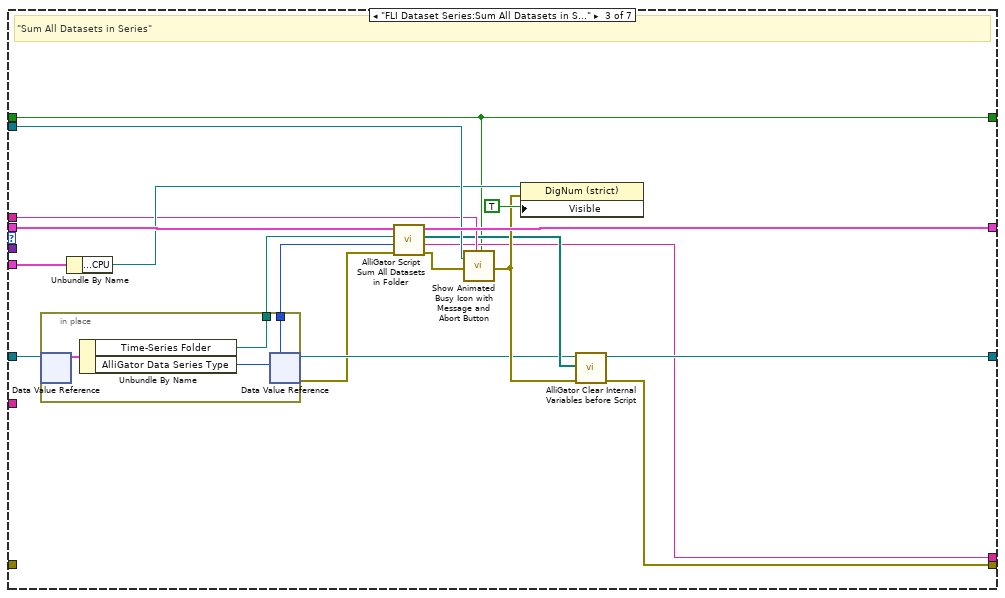
[diagram p3: hidden frame]
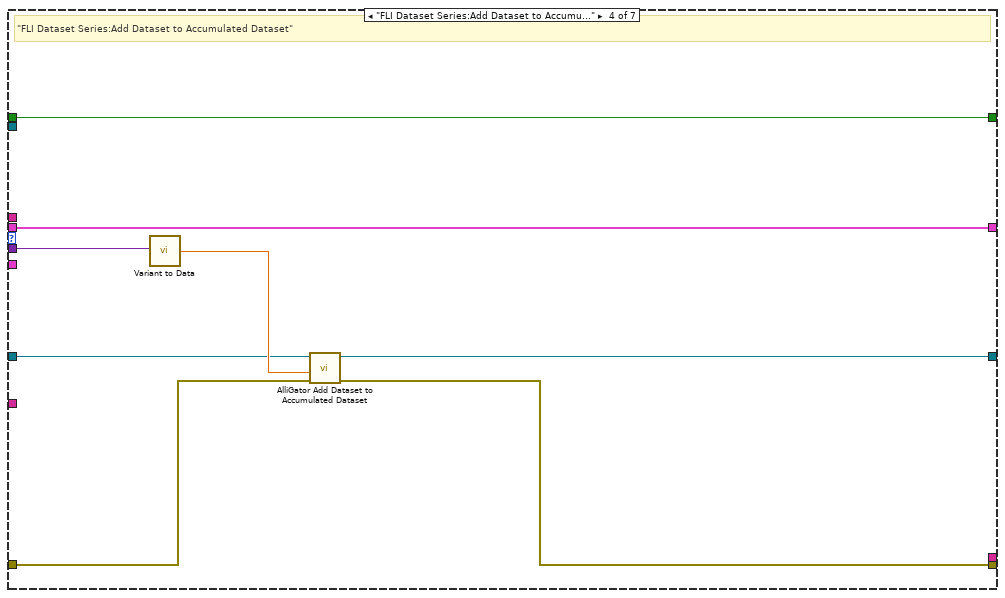
[diagram p4: hidden frame]
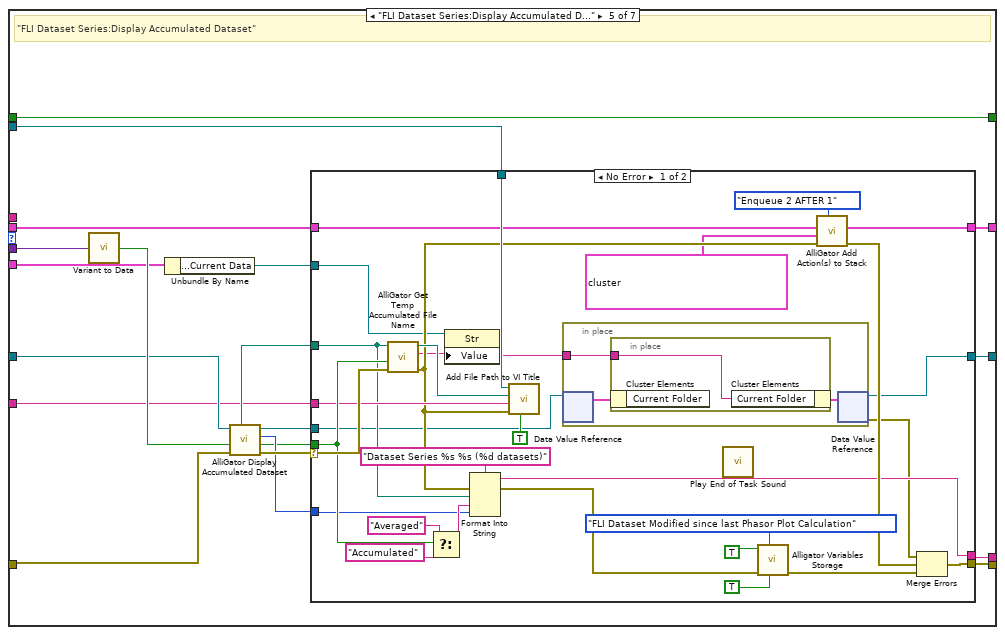
[diagram p5: hidden frame]
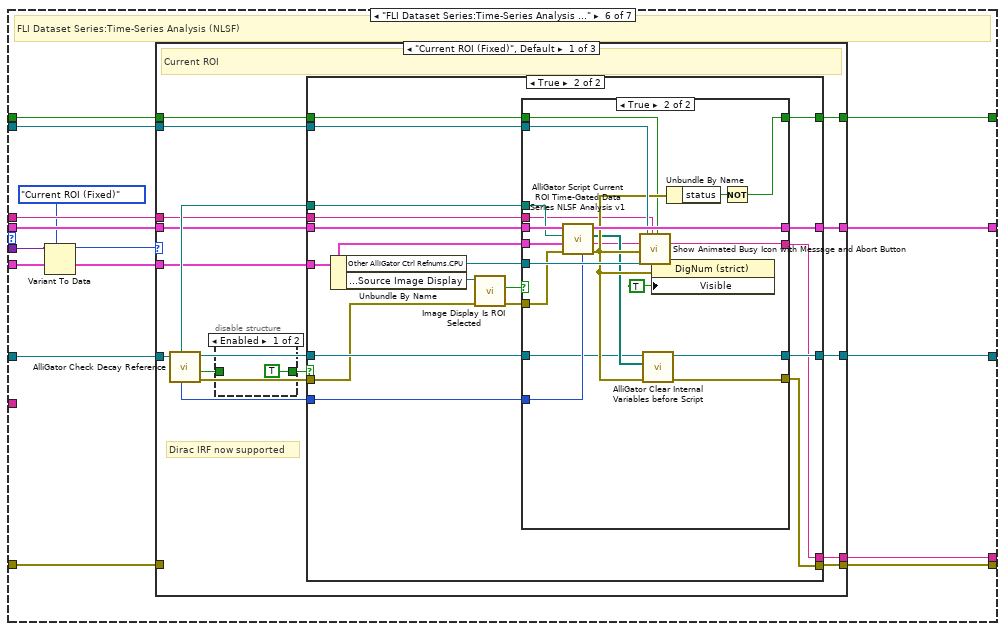
[diagram p7: hidden frame]
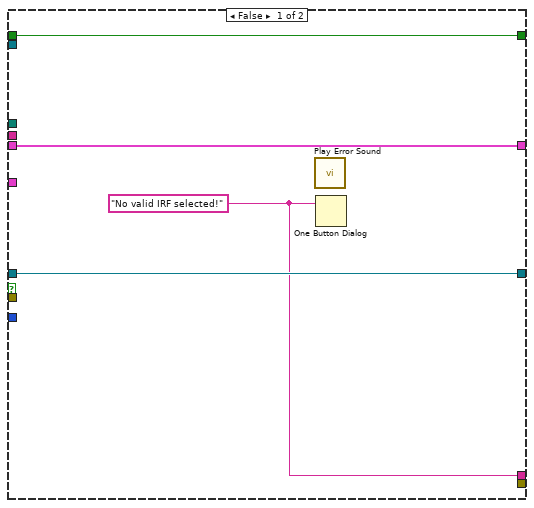
[diagram p9: hidden frame]
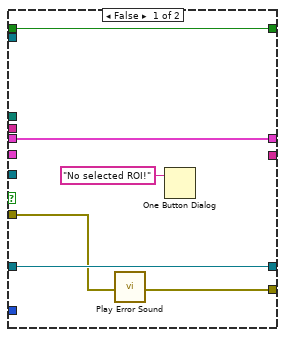
[diagram p10: hidden frame]
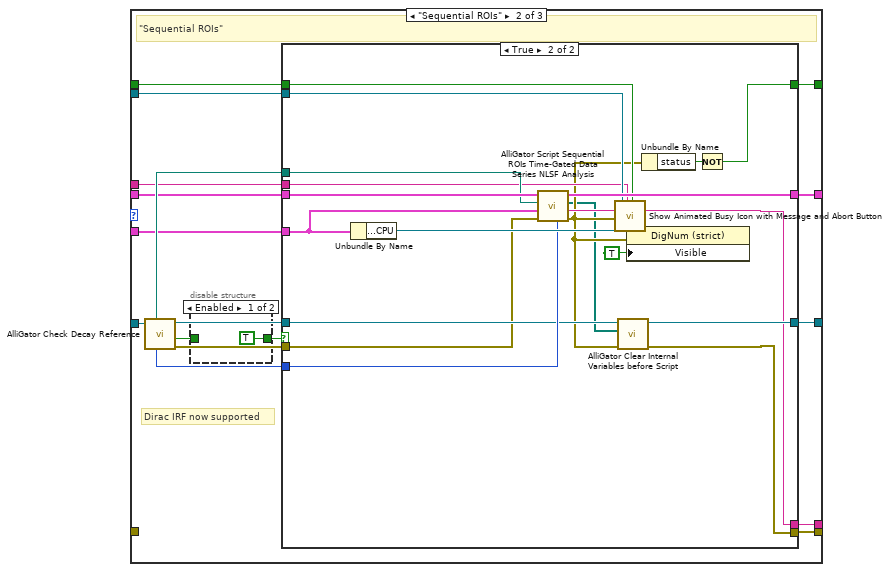
[diagram p11: hidden frame]
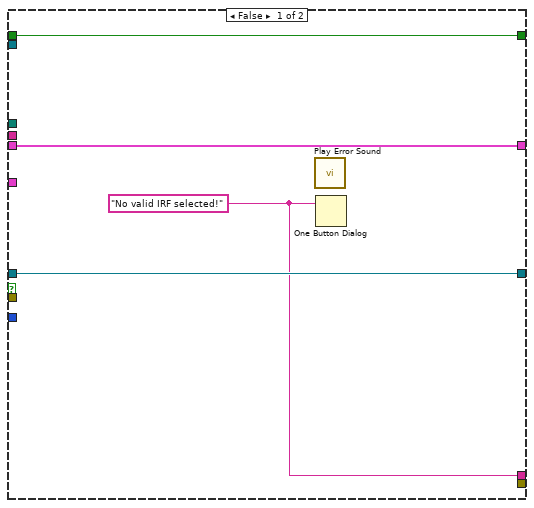
[diagram p13: hidden frame]
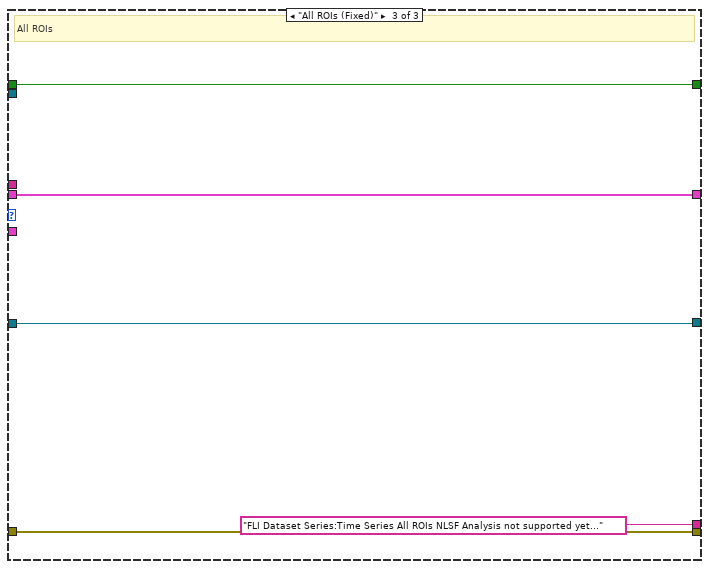
[diagram p14: hidden frame]
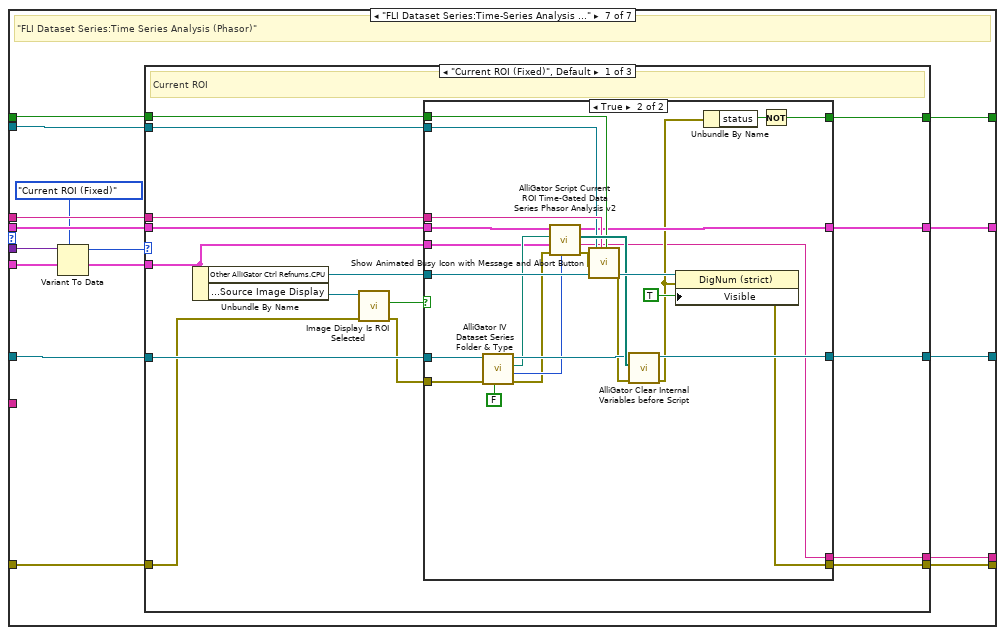
[diagram p15: hidden frame]
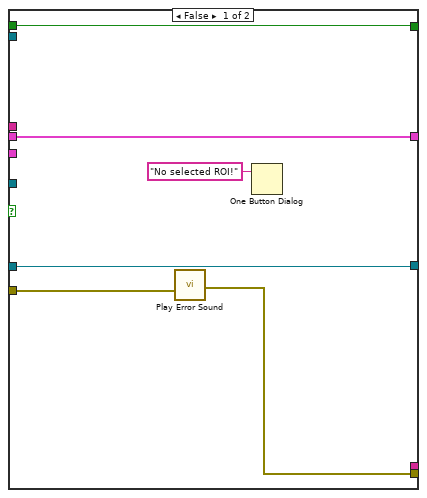
[diagram p16: hidden frame]
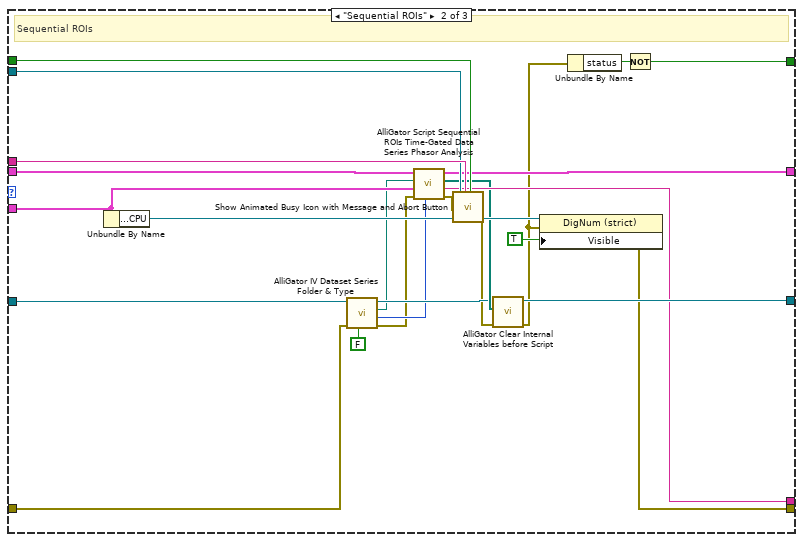
[diagram p17: hidden frame]
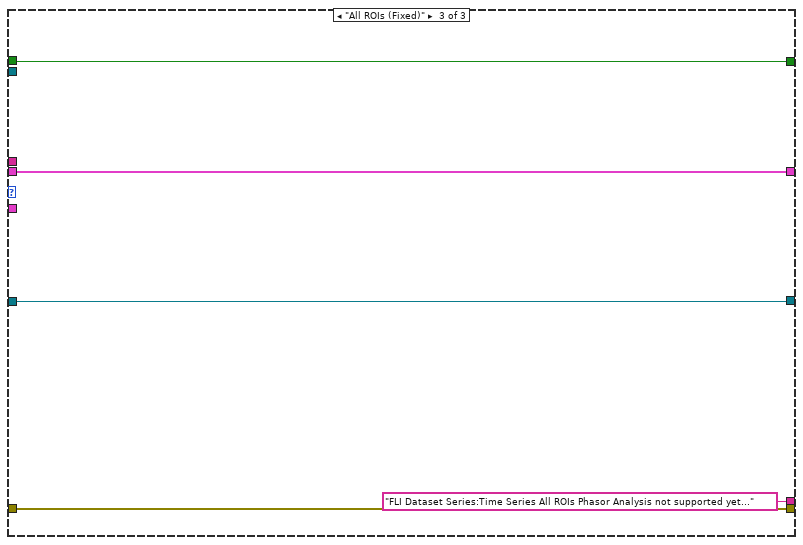
[diagram p18: hidden frame]
diagram:
  # "Author: Xavier Michalet\nCopyright 2025 REGENTS OF THE UNIVERSITY OF CALIFORNIA\n\nRedistribution and use in source and binary forms, with or without modification, are permitted provided that the following conditions are met:\n\n1. Redistributions of source code must retain the above copyright notice, this list of conditions and the following disclaimer.\n\n2. Redistributions in binary form must reproduce the above copyright notice, this list of conditions and the following disclaimer in the documentation and/or other materials provided with the distribution.\n\n3. Neither the name of the copyright holder nor the names of its contributors may be used to endorse or promote products derived from this software without specific prior written permission.\n\nTHIS SOFTWARE IS PROVIDED BY THE COPYRIGHT HOLDERS AND CONTRIBUTORS “AS IS” AND ANY EXPRESS OR IMPLIED WARRANTIES, INCLUDING, BUT NOT LIMITED TO, THE IMPLIED WARRANTIES OF MERCHANTABILITY AND FITNESS FOR A PARTICULAR PURPOSE ARE DISCLAIMED. IN NO EVENT SHALL THE COPYRIGHT HOLDER OR CONTRIBUTORS BE LIABLE FOR ANY DIRECT, INDIRECT, INCIDENTAL, SPECIAL, EXEMPLARY, OR CONSEQUENTIAL DAMAGES (INCLUDING, BUT NOT LIMITED TO, PROCUREMENT OF SUBSTITUTE GOODS OR SERVICES; LOSS OF USE, DATA, OR PROFITS; OR BUSINESS INTERRUPTION) HOWEVER CAUSED AND ON ANY THEORY OF LIABILITY, WHETHER IN CONTRACT, STRICT LIABILITY, OR TORT (INCLUDING NEGLIGENCE OR OTHERWISE) ARISING IN ANY WAY OUT OF THE USE OF THIS SOFTWARE, EVEN IF ADVISED OF THE POSSIBILITY OF SUCH DAMAGE."
  n1 = global read "AlliGator Globals.vi" "Alligator version"() -> (w5:string)
  n2 = call "AlliGator Event to String.vi"("AlliGator Q Event"="AlliGator Q Event in") -> ("String"=w7:string)  [unwired: 8 in]
  n3 = case shown="\"FLI Dataset Series:Clear Dataset Series Sum\"" "AlliGator Q Event in" {
    tunnel: "Data" -> [_ _ _ w62 w73 w124 w252]
    tunnel: "AlliGator Q Elements" -> [w21 w35 w53 w65 w77 w134 w264]
    tunnel: [w21 w35 w54 w65 w76 w129 w255] -> w9
    tunnel: "VI in" -> [_ w34 w51 _ w75 w135 w261]
    tunnel: [w20 w22 w36 w64 w74 w128 w254] -> w10
    tunnel: "Script in" -> [w20 w22 w36 w64 w74 w136 w260]
    tunnel: w7 -> [_ w28 w42 _ _ w127 w263]
    tunnel: "error in (no error)" -> [w19 _ _ w59 w67 w125 w253]
    tunnel: [w19 w33 w43 w60 w66 w131 w256] -> w6
    tunnel: "AlliGator Ctrl Refnums" -> [_ w32 w50 _ w72 w133 w262]
    tunnel: "AlliGator IV DVR in" -> [w18 w27 w39 w61 w71 w132 w259]
    tunnel: [w18 w25 w44 w58 w70 w130 w258] -> w17
    tunnel: [_ w23 w40 _ w68 w126 w257] -> w2
    tunnel: w5 -> [_ _ _ _ w69 _ _]
    frame "---- FLI Dataset Series ----", Default {
    }
    frame "FLI Dataset Series:Clear Dataset Series Sum" {
      w29 = FALSE ("Visible")
      # "\"Clear Dataset Series Sum\""
      n4 = Unbundle By Name(w32) -> ("Dataset Control References.Time Point Slide"=w31:refnum<vi>, "Dataset Control References.Current Data"=w30:refnum<vi>)
      n5 = call "Show Animated Busy Icon with Message.vi"("Already active? (F)"=w22, "Message"=w28, "Target VI Refnum"=w34) -> ("Error Out"=w26:errorcluster)  [unwired: 8 in]
      n6 = call "AlliGator Clear Dataset Series Sum.vi"("error in (no error)"=w26, "Data Value Reference in"=w27) -> ("error out"=w24:errorcluster, "Message"=w23:string, "Data Value Reference out"=w25:refnum<data-value>)  [unwired: 7 in]
      n7 = call "Hide Animated Busy Icon with Message.vi"("Already active? (F)"=w22, "Error In"=w24, "Target VI reference"=w34) -> ("Error Out"=w33:errorcluster)  [unwired: 8 in]
      n8 = property class="Str"(reference=w30, "Visible"=w29) -> ()  [unwired: 1 in, 2 out]
      n9 = property class="Slide (strict)"(reference=w31, error in=w24, "Visible"=w29) -> ()  [unwired: 2 out]
    }
    frame "FLI Dataset Series:Sum All Datasets in Series" {
      # "\"Sum All Datasets in Series\""
      n10 = in-place {
        in-place-border: [w57] -> w46
        in-place-border: [w56] -> w45
        n11 = in-place-dvr #1(w39) -> (w55:T17)  [unwired: 1 out]
        n12 = Unbundle By Name(w55) -> ("Time-Series Folder"=w57:path, "AlliGator Data Series Type"=w56:T21)
        n13 = in-place-dvr #1() -> (w38:refnum<data-value>, w37:errorcluster)  [unwired: 1 in]
      }
      n14 = Unbundle By Name(w50) -> ("Other AlliGator Ctrl Refnums.CPU"=w47:refnum<vi>)
      n15 = call "AlliGator Script Sum All Datasets in Folder.vi"("Error In"=w37, "AlliGator Data Series Type"=w45, "Path"=w46, "Alligator Queue Elements in"=w53) -> ("Error Out"=w52:errorcluster, "Message"=w40:string, "[Time-Series Path]"=w41:path[], "Alligator Queue Elements out"=w54:T4[])  [unwired: 4 in]
      n16 = call "Show Animated Busy Icon with Message and Abort Button.vi"("Already active? (F)"=w36, "Message"=w42, "Target VI reference"=w51, "Error In"=w52) -> ("Error Out"=w48:errorcluster)  [unwired: 15 in]
      n17 = property class="DigNum (strict)"(reference=w47, error in=w48, "Visible"=TRUE) -> ()  [unwired: 2 out]
      n18 = call "AlliGator Clear Internal Variables before Script.vi"("Error In"=w48, "[Time-Series Path]"=w41, "AlliGator Internal Variables DVR in"=w38) -> ("Error Out"=w43:errorcluster, "AlliGator Internal Variables DVR out"=w44:refnum<data-value>)  [unwired: 7 in]
    }
    frame "FLI Dataset Series:Add Dataset to Accumulated Dataset" {
      # "\"FLI Dataset Series:Add Dataset to Accumulated Dataset\""
      n19 = call-poly "Variant to Data.vi"("Variant"=w62) -> ("Value"=w63:dbl)  [unwired: 8 in]
      n20 = call "AlliGator Add Dataset to Accumulated Dataset.vi"("error in (no error)"=w59, "Weight (1)"=w63, "AlliGator IV DVR in"=w61) -> ("error out"=w60:errorcluster, "AlliGator IV DVR out"=w58:refnum<data-value>)  [unwired: 7 in]
    }
    frame "FLI Dataset Series:Display Accumulated Dataset" {
      # "\"FLI Dataset Series:Display Accumulated Dataset\""
      n21 = call-poly "Variant to Data.vi"("Variant"=w73) -> ("Value"=w81:bool)  [unwired: 8 in]
      n22 = Unbundle By Name(w72) -> ("Dataset Control References.Current Data"=w80:refnum<vi>)
      n23 = call "AlliGator Display Accumulated Dataset.vi"("error in (no error)"=w67, "Sum (F) or Average (T)"=w81, "AlliGator IV DVR in"=w71) -> ("error out"=w83:errorcluster, "Averaged?"=w78:bool, "# Accumulated Datasets"=w79:i32, "AlliGator IV DVR out"=w84:refnum<data-value>, "Time-Series Folder"=w82:path)  [unwired: 4 in]
      n24 = case shown="No Error" w83 {
        selector: w83 -> [w112 w121]
        tunnel: w75 -> [w114 _]
        tunnel: w82 -> [w104 _]
        tunnel: [w111 w121] -> w66
        tunnel: w78 -> [w107 _]
        tunnel: w69 -> [w105 _]
        tunnel: w79 -> [w102 _]
        tunnel: w77 -> [w101 w120]
        tunnel: [w100 w120] -> w76
        tunnel: w80 -> [w95 _]
        tunnel: w84 -> [w87 w119]
        tunnel: [w85 w119] -> w70
        tunnel: [w93 _] -> w68
        frame No Error {
          n25 = call "AlliGator Get Temp Accumulated File Name.vi"("error in (no error)"=w112, "Averaged?"=w107, "Time-Series Folder"=w104) -> ("error out"=w99:errorcluster, "filename without extension"=w94:string, "temporary file name"=w103:path)  [unwired: 6 in]
          n26 = Select(t="Averaged" ("string"), s=w107, f="Accumulated" ("string")) -> (s? t:f=w106:string)
          n27 = property class="Str"(reference=w95, "Value"=w94) -> ()  [unwired: 1 in, 2 out]
          n28 = Format Into String(format string="Dataset Series %s %s (%d datasets)" ("initial string"), error in=w99, w104, w106, w102) -> (resulting string=w93:string, error out=w92:errorcluster)  [unwired: 1 in]
          n29 = call "Add File Path to VI Title.vi"("Add Asterisk?"=TRUE, "Error In"=w99, "VI Title"=w105, "File Path"=w103, "VI Refnum"=w114) -> ()  [unwired: 6 in, 1 out]
          n30 = in-place {
            in-place-border: w94 -> [w117]
            n31 = in-place-dvr #2(w87) -> (w116:T17)  [unwired: 1 out]
            n32 = in-place {
              in-place-border: w117 -> [w118]
              n33 = in-place-cluster #3(w116) -> ()  [unwired: 1 out]
              n34 = in-place-cluster #3("Current Folder"=w118) -> (w115:T17)
            }
            n35 = in-place-dvr #2(w115) -> (w85:refnum<data-value>, w86:errorcluster)
          }
          n36 = call "Play End of Task Sound.vi"() -> ()  [unwired: 27 in, 1 out]
          n37 = call "Alligator Variables Storage.vi"("Get(F)/Set"=TRUE, "AlliGator Variable"=AlliGator_Variables_List."FLI Dataset Modified since last Phasor Plot Calculation" ("Alligator Variable"), "Error In"=w92, "Data in"=TRUE) -> ("Error Out"=w91:errorcluster)  [unwired: 5 in, 2 out]
          n38 = call-poly "AlliGator Add Action(s) to Stack.vi"("Elements Order in Action Stack (Default: 2 BEFORE 1)"=Alligator_Elements_Order_in_Action_Stack."Enqueue 2 AFTER 1", "Error In"=w99, "Alligator Queue Element 2"=T4[] [{"AlliGator Q Event"=enum."Image:Image Histogram", "Data"=variant}, {"AlliGator Q Event"=enum."Image:Image Contrast", "Data"=variant}] ("Alligator Atomic Action"), "Alligator Queue Element 1"=w101) -> ("Error Out"=w98:errorcluster, "Alligator Queue Element 1 (+ 2)"=w100:T4[])  [unwired: 6 in]
          n39 = Merge Errors(w86, w98, w91) -> (w111:errorcluster)
        }
        frame Error {
        }
      }
    }
    frame "FLI Dataset Series:Time-Series Analysis (NLSF)" {
      # "FLI Dataset Series:Time-Series Analysis (NLSF)"
      n40 = Variant To Data(type=AlliGator_Series_Analysis_Type."Current ROI (Fixed)" ("Series Analysis Type"), Variant=w124) -> (data=w122:T16)  [unwired: 1 in, 1 out]
      n41 = case shown="\"Current ROI (Fixed)\", Default" w122 {
        tunnel: w136 -> [w149 w215 w249]
        tunnel: w135 -> [w148 w214 _]
        tunnel: w134 -> [w147 w213 w248]
        tunnel: w133 -> [w146 w212 _]
        tunnel: w132 -> [w145 w211 w247]
        tunnel: [w144 w210 w246] -> w131
        tunnel: [w143 w209 w247] -> w130
        tunnel: [w142 w208 w248] -> w129
        tunnel: [w141 w207 w249] -> w128
        tunnel: w127 -> [w140 w206 _]
        tunnel: [w139 w205 "FLI Dataset Series:Time Series All ROIs NLSF Analysis not supported yet..." ("Message")] -> w126
        tunnel: w125 -> [_ _ w246]
        frame "Current ROI (Fixed)", Default {
          # "Dirac IRF now supported"
          # "Current ROI"
          n42 = call "AlliGator Check Decay Reference.vi"("AlliGator Internal Variables DVR"=w145) -> ("Error Out"=w150:errorcluster, "Valid Reference?"=w138:bool, "AlliGator Internal Variables DVR"=w151:refnum<data-value>, "AlliGator Data Series Type"=w152:T21, "Time-Series Folder"=w153:path)  [unwired: 3 in, 3 out]
          n43 = disable-structure shown="Enabled" {
            disable-tunnel: w138 -> [_ w155]
            disable-tunnel: [TRUE ("Valid Reference?") w155] -> w137
            frame Enabled {
            }
            frame Disabled {
            }
          }
          n44 = case shown="True" w137 {
            tunnel: [w159 w177] -> w142
            tunnel: [_ w171] -> w144
            tunnel: w147 -> [w159 w176]
            tunnel: w149 -> [w158 w166]
            tunnel: [w158 w175] -> w141
            tunnel: w146 -> [_ w160]
            tunnel: w150 -> [_ w163]
            tunnel: w148 -> [_ w174]
            tunnel: [w157 w172] -> w143
            tunnel: w153 -> [_ w170]
            tunnel: w152 -> [_ w169]
            tunnel: w151 -> [w157 w168]
            tunnel: w140 -> [_ w167]
            tunnel: [w156 w165] -> w139
            frame False {
              w156 = "No valid IRF selected!" ("Script Message")
              n45 = call "Play Error Sound.vi"() -> ()  [unwired: 27 in, 1 out]
              n46 = One Button Dialog(message=w156) -> ()  [unwired: 1 in, 1 out]
            }
            frame True {
              n47 = Unbundle By Name(w160) -> ("Other AlliGator Ctrl Refnums.CPU"=w173:refnum<vi>, "Registered Events Ctrl Refnums.Source Image Display"=w164:refnum<vi>)
              n48 = call "Image Display Is ROI Selected.vi"("Error In"=w163, "Image Control Refnum"=w164) -> ("Error Out"=w162:errorcluster, "Is ROI Selected?"=w161:bool)  [unwired: 7 in, 1 out]
              n49 = case shown="True" w161 {
                tunnel: [w183 w202] -> w177
                tunnel: w176 -> [w183 w201]
                tunnel: [w179 w199] -> w175
                tunnel: w174 -> [_ w198]
                tunnel: w173 -> [_ w197]
                tunnel: [w182 w193] -> w172
                tunnel: [w180 w192] -> w171
                tunnel: w170 -> [_ w191]
                tunnel: w169 -> [_ w190]
                tunnel: w168 -> [w182 w189]
                tunnel: w167 -> [_ w188]
                tunnel: w166 -> [w179 w187]
                tunnel: [_ w186] -> w165
                tunnel: w162 -> [w181 w185]
                tunnel: w160 -> [_ w184]
                frame False {
                  n50 = call "Play Error Sound.vi"("Error In"=w181) -> ("Error Out"=w180:errorcluster)  [unwired: 26 in]
                  n51 = One Button Dialog(message="No selected ROI!") -> ()  [unwired: 1 in, 1 out]
                }
                frame True {
                  n52 = call "AlliGator Script Current ROI Time-Gated Data Series NLSF Analysis v1.vi"("AlliGator Data Series Type"=w190, "Error In"=w185, "AlliGator Ctrl Refnums"=w184, "Path"=w191, "Alligator Queue Elements in"=w201) -> ("Error Out"=w196:errorcluster, "Message"=w186:string, "Time-Series Paths"=w194:path[], "Alligator Queue Elements out"=w202:T4[])  [unwired: 3 in]
                  n53 = call "Show Animated Busy Icon with Message and Abort Button.vi"("Already active? (F)"=w187, "Message"=w188, "Target VI reference"=w198, "Error In"=w196) -> ()  [unwired: 15 in, 1 out]
                  n54 = call "AlliGator Clear Internal Variables before Script.vi"("Error In"=w196, "[Time-Series Path]"=w194, "AlliGator Internal Variables DVR in"=w189) -> ("Error Out"=w192:errorcluster, "AlliGator Internal Variables DVR out"=w193:refnum<data-value>)  [unwired: 7 in]
                  n55 = property class="DigNum (strict)"(reference=w197, error in=w196, "Visible"=TRUE) -> ()  [unwired: 2 out]
                  n56 = Unbundle By Name(w196) -> ("status"=w200:bool)
                  n57 = Not(x=w200) -> (.not. x?=w199:bool)
                }
              }
            }
          }
        }
        frame "Sequential ROIs" {
          # "Dirac IRF now supported"
          # "\"Sequential ROIs\""
          n58 = call "AlliGator Check Decay Reference.vi"("AlliGator Internal Variables DVR"=w211) -> ("Error Out"=w216:errorcluster, "Valid Reference?"=w204:bool, "AlliGator Internal Variables DVR"=w217:refnum<data-value>, "AlliGator Data Series Type"=w218:T21, "Time-Series Folder"=w219:path)  [unwired: 3 in, 3 out]
          n59 = disable-structure shown="Enabled" {
            disable-tunnel: w204 -> [_ w221]
            disable-tunnel: [TRUE ("Valid Reference?") w221] -> w203
            frame Enabled {
            }
            frame Disabled {
            }
          }
          n60 = case shown="True" w203 {
            tunnel: [w225 w244] -> w208
            tunnel: [_ w238] -> w210
            tunnel: w213 -> [w225 w243]
            tunnel: w215 -> [w224 w233]
            tunnel: [w224 w242] -> w207
            tunnel: w212 -> [_ w231]
            tunnel: w216 -> [_ w230]
            tunnel: w214 -> [_ w241]
            tunnel: [w223 w239] -> w209
            tunnel: w219 -> [_ w237]
            tunnel: w218 -> [_ w236]
            tunnel: w217 -> [w223 w235]
            tunnel: w206 -> [_ w234]
            tunnel: [w222 w232] -> w205
            frame False {
              w222 = "No valid IRF selected!" ("Script Message")
              n61 = call "Play Error Sound.vi"() -> ()  [unwired: 27 in, 1 out]
              n62 = One Button Dialog(message=w222) -> ()  [unwired: 1 in, 1 out]
            }
            frame True {
              n63 = Unbundle By Name(w231) -> ("Other AlliGator Ctrl Refnums.CPU"=w240:refnum<vi>)
              n64 = call "AlliGator Script Sequential ROIs Time-Gated Data Series NLSF Analysis.vi"("AlliGator Data Series Type"=w236, "Error In"=w230, "AlliGator Ctrl Refnums"=w231, "Path"=w237, "Alligator Queue Elements in"=w243) -> ("Error Out"=w228:errorcluster, "Message"=w232:string, "Time-Series Paths"=w226:path[], "Alligator Queue Elements out"=w244:T4[])  [unwired: 3 in]
              n65 = call "Show Animated Busy Icon with Message and Abort Button.vi"("Already active? (F)"=w233, "Message"=w234, "Target VI reference"=w241, "Error In"=w228) -> ()  [unwired: 15 in, 1 out]
              n66 = call "AlliGator Clear Internal Variables before Script.vi"("Error In"=w228, "[Time-Series Path]"=w226, "AlliGator Internal Variables DVR in"=w235) -> ("Error Out"=w238:errorcluster, "AlliGator Internal Variables DVR out"=w239:refnum<data-value>)  [unwired: 7 in]
              n67 = property class="DigNum (strict)"(reference=w240, error in=w228, "Visible"=TRUE) -> ()  [unwired: 2 out]
              n68 = Unbundle By Name(w228) -> ("status"=w229:bool)
              n69 = Not(x=w229) -> (.not. x?=w242:bool)
            }
          }
        }
        frame "All ROIs (Fixed)" {
          # "All ROIs"
        }
      }
    }
    frame "FLI Dataset Series:Time-Series Analysis (Phasor)" {
      # "\"FLI Dataset Series:Time Series Analysis (Phasor)\""
      n70 = Variant To Data(type=AlliGator_Series_Analysis_Type."Current ROI (Fixed)" ("Series Analysis Type"), Variant=w252) -> (data=w250:T16)  [unwired: 1 in, 1 out]
      n71 = case shown="\"Current ROI (Fixed)\", Default" w250 {
        tunnel: w264 -> [w279 w333 w338]
        tunnel: w263 -> [w278 w332 _]
        tunnel: w262 -> [w265 w322 _]
        tunnel: w261 -> [w277 w331 _]
        tunnel: w260 -> [w276 w330 w339]
        tunnel: w259 -> [w275 w329 w337]
        tunnel: [w274 w328 w337] -> w258
        tunnel: [w273 w327 "FLI Dataset Series:Time Series All ROIs Phasor Analysis not supported yet..." ("Message")] -> w257
        tunnel: [w272 w326 w336] -> w256
        tunnel: [w271 w325 w338] -> w255
        tunnel: [w270 w324 w339] -> w254
        tunnel: w253 -> [w268 w323 w336]
        frame "Current ROI (Fixed)", Default {
          # "Current ROI"
          n72 = Unbundle By Name(w265) -> ("Other AlliGator Ctrl Refnums.CPU"=w280:refnum<vi>, "Registered Events Ctrl Refnums.Source Image Display"=w269:refnum<vi>)
          n73 = call "Image Display Is ROI Selected.vi"("Error In"=w268, "Image Control Refnum"=w269) -> ("Error Out"=w267:errorcluster, "Is ROI Selected?"=w266:bool)  [unwired: 7 in, 1 out]
          n74 = case shown="True" w266 {
            tunnel: w280 -> [_ w308]
            tunnel: w279 -> [w285 w300]
            tunnel: w278 -> [_ w299]
            tunnel: w277 -> [_ w298]
            tunnel: w276 -> [w286 w297]
            tunnel: w275 -> [w284 w296]
            tunnel: [w284 w295] -> w274
            tunnel: [_ w289] -> w273
            tunnel: [w281 w294] -> w272
            tunnel: [w285 w293] -> w271
            tunnel: [w286 w291] -> w270
            tunnel: w267 -> [w282 w287]
            tunnel: w265 -> [_ w288]
            frame False {
              n75 = call "Play Error Sound.vi"("Error In"=w282) -> ("Error Out"=w281:errorcluster)  [unwired: 26 in]
              n76 = One Button Dialog(message="No selected ROI!") -> ()  [unwired: 1 in, 1 out]
            }
            frame True {
              n77 = call "AlliGator IV Dataset Series Folder & Type.vi"("Get (F)/ Set (T)"=FALSE, "error in (no error)"=w287, "AlliGator IV DVR in"=w296) -> ("error out"=w302:errorcluster, "AlliGator Data Series Type"=w303:T21, "Time-Series Folder"=w304:path, "AlliGator IV DVR out"=w305:refnum<data-value>)  [unwired: 4 in, 1 out]
              n78 = call "AlliGator Script Current ROI Time-Gated Data Series Phasor Analysis v2.vi"("AlliGator Data Series Type"=w303, "Error In"=w302, "AlliGator Ctrl Refnums"=w288, "Path"=w304, "Alligator Queue Elements in"=w300) -> ("Error Out"=w309:errorcluster, "Message"=w289:string, "Time-Series Paths"=w306:path[], "Alligator Queue Elements out"=w293:T4[])  [unwired: 3 in]
              n79 = call "Show Animated Busy Icon with Message and Abort Button.vi"("Already active? (F)"=w297, "Message"=w299, "Target VI reference"=w298, "Error In"=w309) -> ("Error Out"=w292:errorcluster)  [unwired: 15 in]
              n80 = call "AlliGator Clear Internal Variables before Script.vi"("Error In"=w292, "[Time-Series Path]"=w306, "AlliGator Internal Variables DVR in"=w305) -> ("Error Out"=w290:errorcluster, "AlliGator Internal Variables DVR out"=w295:refnum<data-value>)  [unwired: 7 in]
              n81 = property class="DigNum (strict)"(reference=w308, error in=w290, "Visible"=TRUE) -> (error out=w294:errorcluster)  [unwired: 1 out]
              n82 = Unbundle By Name(w290) -> ("status"=w310:bool)
              n83 = Not(x=w310) -> (.not. x?=w291:bool)
            }
          }
        }
        frame "Sequential ROIs" {
          # "Sequential ROIs"
          n84 = Unbundle By Name(w322) -> ("Other AlliGator Ctrl Refnums.CPU"=w334:refnum<vi>)
          n85 = call "AlliGator IV Dataset Series Folder & Type.vi"("Get (F)/ Set (T)"=FALSE, "error in (no error)"=w323, "AlliGator IV DVR in"=w329) -> ("error out"=w314:errorcluster, "AlliGator Data Series Type"=w315:T21, "Time-Series Folder"=w316:path, "AlliGator IV DVR out"=w317:refnum<data-value>)  [unwired: 4 in, 1 out]
          n86 = call "AlliGator Script Sequential ROIs Time-Gated Data Series Phasor Analysis.vi"("AlliGator Data Series Type"=w315, "Error In"=w314, "AlliGator Ctrl Refnums"=w322, "Path"=w316, "Alligator Queue Elements in"=w333) -> ("Error Out"=w320:errorcluster, "Message"=w327:string, "Time-Series Paths"=w318:path[], "Alligator Queue Elements out"=w325:T4[])  [unwired: 3 in]
          n87 = call "Show Animated Busy Icon with Message and Abort Button.vi"("Already active? (F)"=w330, "Message"=w332, "Target VI reference"=w331, "Error In"=w320) -> ("Error Out"=w312:errorcluster)  [unwired: 15 in]
          n88 = call "AlliGator Clear Internal Variables before Script.vi"("Error In"=w312, "[Time-Series Path]"=w318, "AlliGator Internal Variables DVR in"=w317) -> ("Error Out"=w311:errorcluster, "AlliGator Internal Variables DVR out"=w328:refnum<data-value>)  [unwired: 7 in]
          n89 = property class="DigNum (strict)"(reference=w334, error in=w311, "Visible"=TRUE) -> (error out=w326:errorcluster)  [unwired: 1 out]
          n90 = Unbundle By Name(w311) -> ("status"=w321:bool)
          n91 = Not(x=w321) -> (.not. x?=w324:bool)
        }
        frame "All ROIs (Fixed)" {
        }
      }
    }
  }
  "AlliGator IV DVR out" <- w17
  "error out" <- w6
  "Script out" <- w10
  "Alligator Queue Elements" <- w9
  n92 = call "Result Style.vi"() -> ("Default Text Formatting"=w1:T2)
  n93 = call "AlliGator Package Notebook Messages.vi"("Message Formatting"=w1, "Message"=w2, "AlliGator Q Event in"="AlliGator Q Event in") -> ("[Notebook Message]"=→"[Notebook Message]":T1[])  [unwired: 8 in]
